vi "Traffic Lights Simulation.vi"() -> ()   [LabVIEW 2024]
panel:
  in  "Day_time":dbl
  out "Green":bool
  out "Yellow":bool
  out "Red":bool
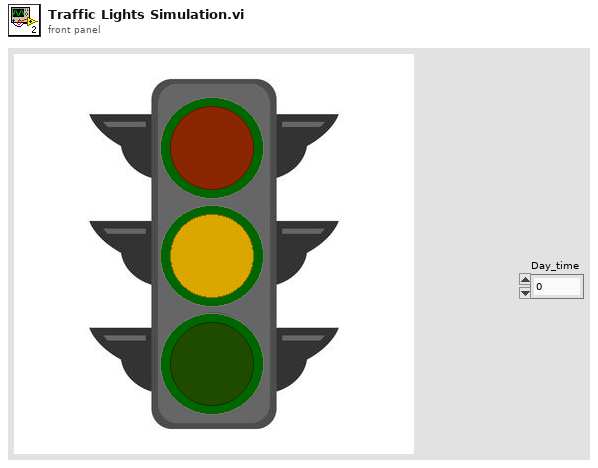
[diagram p1: front panel]
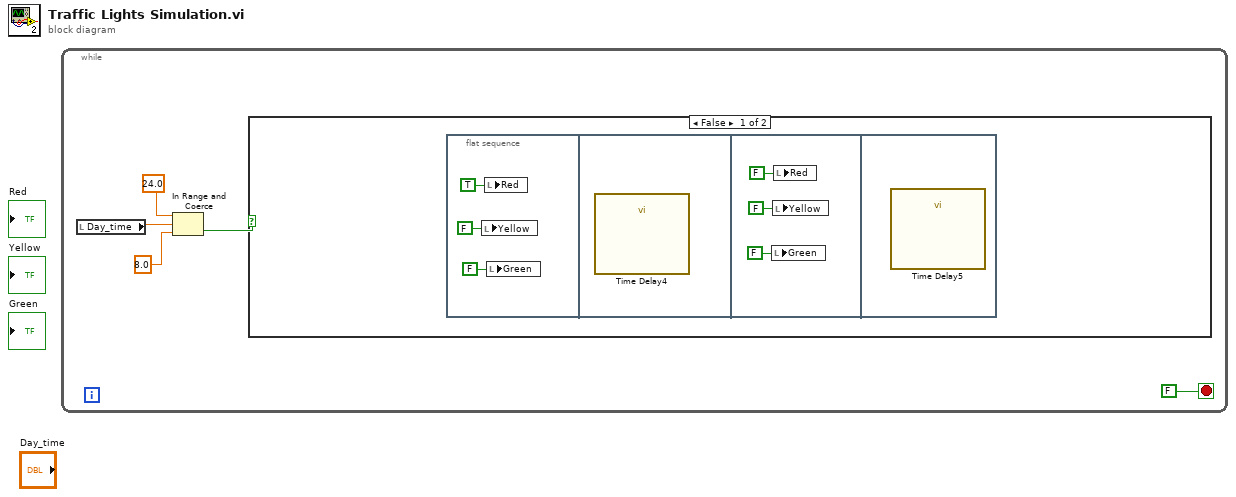
[diagram p0: block diagram]
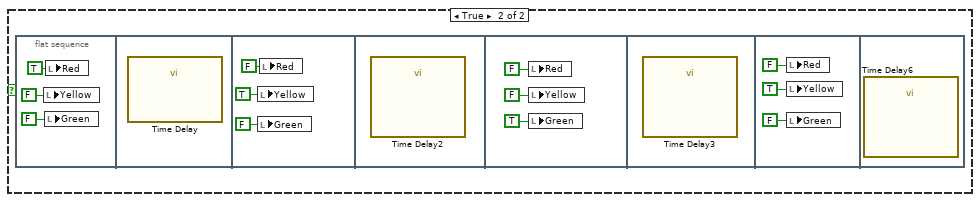
[diagram p2: hidden frame]
diagram:
  n1 = while {
    stop <- FALSE stop-if-true
    n2 = local read "Day_time"() -> (w2:dbl)
    n3 = In Range and Coerce(upper limit=24.0, x=w2, lower limit=8.0) -> (In Range?=w1:bool)  [unwired: 1 out]
    n4 = case shown="False" w1 {
      frame False {
        n5 = flat-sequence {
          frame #0 {
            n6 = local write "Yellow"(FALSE ("Yellow")) -> ()
            n7 = local write "Red"(TRUE ("Red")) -> ()
            n8 = local write "Green"(FALSE ("Green")) -> ()
          }
          frame #1 {
            n9 = call "Time Delay4"() -> ()  [unwired: 11 in, 1 out]
          }
          frame #2 {
            n10 = local write "Green"(FALSE ("Green")) -> ()
            n11 = local write "Yellow"(FALSE ("Yellow")) -> ()
            n12 = local write "Red"(FALSE ("Red")) -> ()
          }
          frame #3 {
            n13 = call "Time Delay5"() -> ()  [unwired: 11 in, 1 out]
          }
        }
      }
      frame True {
        n14 = flat-sequence {
          frame #0 {
            n15 = local write "Yellow"(FALSE ("Yellow")) -> ()
            n16 = local write "Green"(FALSE ("Green")) -> ()
            n17 = local write "Red"(TRUE ("Red")) -> ()
          }
          frame #1 {
            n18 = call "Time Delay"() -> ()  [unwired: 11 in, 1 out]
          }
          frame #2 {
            n19 = local write "Yellow"(TRUE ("Yellow")) -> ()
            n20 = local write "Green"(FALSE ("Green")) -> ()
            n21 = local write "Red"(FALSE ("Red")) -> ()
          }
          frame #3 {
            n22 = call "Time Delay2"() -> ()  [unwired: 11 in, 1 out]
          }
          frame #4 {
            n23 = local write "Red"(FALSE ("Red")) -> ()
            n24 = local write "Yellow"(FALSE ("Yellow")) -> ()
            n25 = local write "Green"(TRUE ("Green")) -> ()
          }
          frame #5 {
            n26 = call "Time Delay3"() -> ()  [unwired: 11 in, 1 out]
          }
          frame #6 {
            n27 = local write "Red"(FALSE ("Red")) -> ()
            n28 = local write "Yellow"(TRUE ("Yellow")) -> ()
            n29 = local write "Green"(FALSE ("Green")) -> ()
          }
          frame #7 {
            n30 = call "Time Delay6"() -> ()  [unwired: 11 in, 1 out]
          }
        }
      }
    }
  }
